vi "set app font.vi"(8 "font size":u32=15, 9 "font name (App Font)":string="App Font", 10 "make lower case":bool, 11 "vis":refnum<vi>[](array[refnum])) -> (0 "error report":errorcluster[](array[cluster]))   [LabVIEW 2013, in "control label adjustment.lvclass"]
uses:
  control label adjustment.lvclass
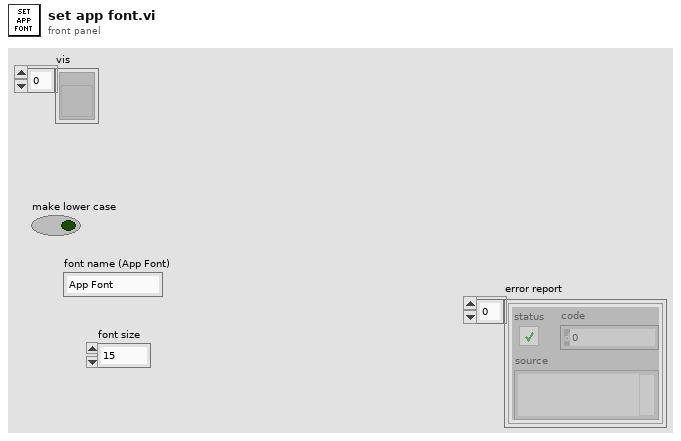
[diagram p1: front panel]
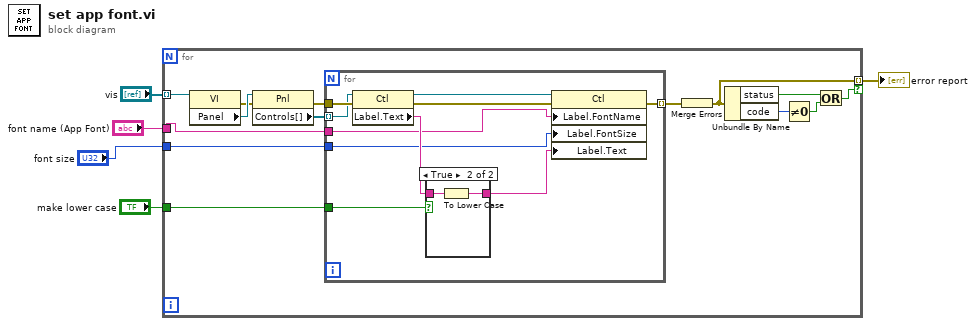
[diagram p0: block diagram]
diagram:
  n1 = for {
    tunnel: "vis" -> [w19] mode=indexing
    tunnel: [w9] -> w4 mode=indexing if=w15
    tunnel: "make lower case" -> [w8]
    tunnel: "font size" -> [w7]
    tunnel: "font name (App Font)" -> [w6]
    n2 = property class="VI"(reference=w19) -> (error out=w10:errorcluster, "Panel"=w14:refnum<vi>)  [unwired: 1 in, 1 out]
    n3 = property class="Pnl"(reference=w14, error in=w10) -> (error out=w12:errorcluster, "Controls[]"=w13:refnum<vi>[])  [unwired: 1 out]
    n4 = for {
      tunnel: w13 -> [w26] mode=indexing
      tunnel: [w29] -> w11 mode=indexing
      tunnel: w12 -> [w28]
      tunnel: w8 -> [w22]
      tunnel: w7 -> [w21]
      tunnel: w6 -> [w20]
      n5 = property class="Ctl"(reference=w26, error in=w28) -> (reference out=w25:refnum<vi>, error out=w27:errorcluster, "Label.Text"=w24:string)
      n6 = case shown="True" w22 {
        tunnel: w24 -> [w30 w32]
        tunnel: [w30 w31] -> w23
        frame False {
        }
        frame True {
          n7 = To Lower Case(string=w32) -> (all lower case string=w31:string)
        }
      }
      n8 = property class="Ctl"(reference=w25, error in=w27, "Label.FontName"=w20, "Label.FontSize"=w21, "Label.Text"=w23) -> (error out=w29:errorcluster)  [unwired: 1 out]
    }
    n9 = Merge Errors(w11) -> (w9:errorcluster)
    n10 = Unbundle By Name(w9) -> ("status"=w18:bool, "code"=w17:i32)
    n11 = Not Equal To 0?(x=w17) -> (x != 0?=w16:bool)
    n12 = Or(x=w18, y=w16) -> (x .or. y?=w15:bool)
  }
  "error report" <- w4
